vi "FL Generate 3D Graph.vi"(0 "Fuzzy Set In":T1 {"user MF interpolating polynomials"."coa_x(y) coeff" format="%.4g"; "user MF interpolating polynomials"."Area(y) coeff" format="%.4g"; "user MF interpolating polynomials"."X(y) coeff" format="%.4g"; "user MF interpolating polynomials"."Y(x) coeff" format="%.4g"; "user MF interpolating polynomials"."Y" format="%.4g"; "user MF interpolating polynomials"."X" format="%.4g"; "defuzzification method" items=["Center of Area", "Modified Center of Area", "Center of Sums", "Center of Maximum", "Mean of Maximum"]; "rules"."consequents"."Var Index" min=0; "rules"."consequents"."Cond" items=["=", "!="]; "rules"."consequents"."MF Index" min=0; "rules"."antecedents"."Var Index" min=0; "rules"."antecedents"."Cond" items=["=", "!="]; "rules"."antecedents"."MF Index" min=0; "rules"."consequent implication" items=["Minimum", "Product"]; "rules"."antecedent connective" items=["AND (Minimum)", "AND (Product)", "OR (Maximum)", "OR (Probabilistic)"]; "output variables"."MFs"."shape" items=["Triangle", "Trapezoid", "Singleton", "Sigmoid", "Gaussian", "User-Defined"]; "input variables"."MFs"."shape" items=["Triangle", "Trapezoid", "Singleton", "Sigmoid", "Gaussian", "User-Defined"]}, 1 "Input":dbl[](array[numeric]), 5 "Input Selection 1":i32, 7 "Input Selection 2":i32=1, 9 "Output":i32, 11 "error in (no error)":errorcluster, 12 "number of samples 1":i32=20, 13 "number of samples 2":i32=20) -> (4 "x":dbl[](array[numeric]), 6 "y":dbl[](array[numeric]), 10 "z":dbl[][](array[numeric]), 15 "error out":errorcluster)   [LabVIEW 2017, in "NI_Fuzzy_Logic_API.lvlib"]
uses:
  <vilib>/addons/Fuzzy Logic/NI_Fuzzy_Logic_API.lvlib
  <vilib>/addons/Fuzzy Logic/TypeDefs/FL System.ctl
  <vilib>/addons/Fuzzy Logic/TypeDefs/FL Variable.ctl
  <vilib>/addons/Fuzzy Logic/TypeDefs/FL Membership Function.ctl
  <vilib>/addons/Fuzzy Logic/TypeDefs/FL Membership Function Shape.ctl
  <vilib>/addons/Fuzzy Logic/TypeDefs/FL Rule.ctl
  <vilib>/addons/Fuzzy Logic/TypeDefs/FL Antecedent.ctl
  <vilib>/addons/Fuzzy Logic/TypeDefs/FL Modifier.ctl
  <vilib>/addons/Fuzzy Logic/TypeDefs/FL Antecedent Connective.ctl
  <vilib>/addons/Fuzzy Logic/TypeDefs/FL Consequent.ctl
  <vilib>/addons/Fuzzy Logic/TypeDefs/FL Consequent Implication.ctl
  <vilib>/addons/Fuzzy Logic/TypeDefs/FL Defuzzification.ctl
  <vilib>/addons/Fuzzy Logic/TypeDefs/FL Interpolating polynomials.ctl
  <vilib>/Analysis/1siggen.llb/Ramp Pattern by Samples.vi
  <vilib>/addons/Fuzzy Logic/FL Fuzzy Controller (MIMO).vi
  <vilib>/Analysis/NI_AALBase.lvlib
panel:
  # "IF"
  # "THEN"
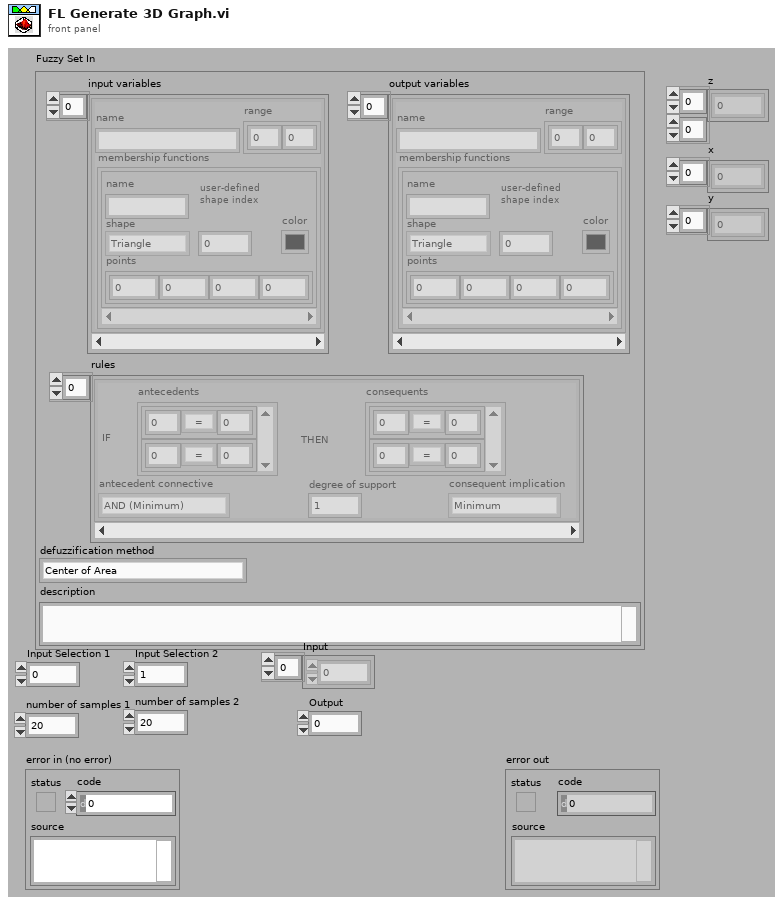
[diagram p1: front panel]
types:
  T1 = typedef "NI_Fuzzy_Logic_API.lvlib/FL System.ctl" = cluster{"input variables":T2[], "output variables":T2[], "rules":T5[], "defuzzification method":T11, "description":string, "user MF interpolating polynomials":T12[]}
  T2 = typedef "NI_Fuzzy_Logic_API.lvlib/FL Variable.ctl" = cluster{"name":string, "range":dbl[], "MFs":T3[]}
  T3 = typedef "NI_Fuzzy_Logic_API.lvlib/FL Membership Function.ctl" = cluster{"name":string, "shape":T4, "points":dbl[], "color":u32, "user-defined shape index":i32}
  T4 = typedef "NI_Fuzzy_Logic_API.lvlib/FL Membership Function Shape.ctl" = u16
  T5 = typedef "NI_Fuzzy_Logic_API.lvlib/FL Rule.ctl" = cluster{"antecedents":T6[], "antecedent connective":T8, "consequents":T9[], "consequent implication":T10, "degree of support":dbl}
  T6 = typedef "NI_Fuzzy_Logic_API.lvlib/FL Antecedent.ctl" = cluster{"Var Index":i32, "MF Index":i32, "Cond":T7}
  T7 = typedef "NI_Fuzzy_Logic_API.lvlib/FL Modifier.ctl" = u16
  T8 = typedef "NI_Fuzzy_Logic_API.lvlib/FL Antecedent Connective.ctl" = u16
  T9 = typedef "NI_Fuzzy_Logic_API.lvlib/FL Consequent.ctl" = cluster{"Var Index":i32, "MF Index":i32, "Cond":T7}
  T10 = typedef "NI_Fuzzy_Logic_API.lvlib/FL Consequent Implication.ctl" = u16
  T11 = typedef "NI_Fuzzy_Logic_API.lvlib/FL Defuzzification.ctl" = u16
  T12 = typedef "NI_Fuzzy_Logic_API.lvlib/FL Interpolating polynomials.ctl" = cluster{"X":dbl[], "Y":dbl[], "Y(x) coeff":dbl[][], "X(y) coeff":dbl[][], "Area(y) coeff":dbl[][], "coa_x(y) coeff":dbl[][]}
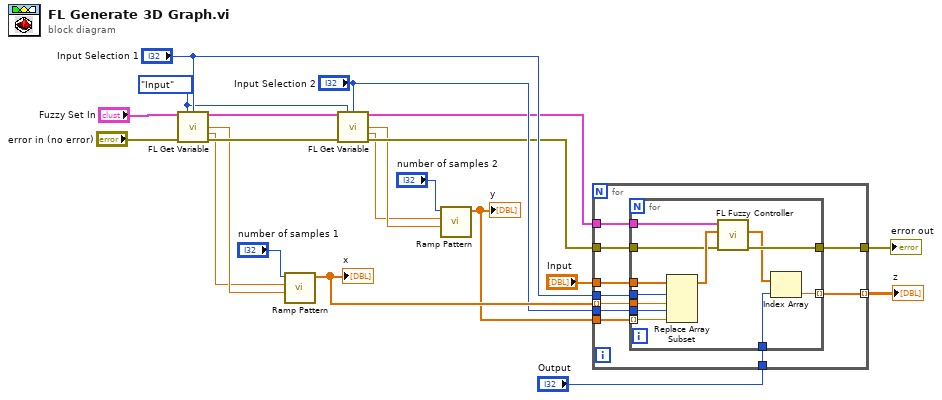
[diagram p0: block diagram]
diagram:
  w8 = enum16{"Input", "Output"}."Input" ("Input/Output")
  n1 = call <vilib>:"FL Get Variable.vi"("fuzzy system in"="Fuzzy Set In", "input/output"=w8, "variable index"="Input Selection 1", "error in (no error)"="error in (no error)") -> ("fuzzy system out"=w11:T1, "minimum"=w4:dbl, "maximum"=w3:dbl, "error out"=w9:errorcluster)  [unwired: 8 out]
  n2 = call-poly <vilib>:"Ramp Pattern.vi"("start"=w4, "end"=w3, "samples"="number of samples 1") -> ("Ramp Pattern"=w19:dbl[])  [unwired: 7 in, 1 out]
  "x" <- w19
  n3 = call <vilib>:"FL Get Variable.vi"("fuzzy system in"=w11, "input/output"=w8, "variable index"="Input Selection 2", "error in (no error)"=w9) -> ("fuzzy system out"=w10:T1, "minimum"=w2:dbl, "maximum"=w1:dbl, "error out"=w6:errorcluster)  [unwired: 8 out]
  n4 = call-poly <vilib>:"Ramp Pattern.vi"("start"=w2, "end"=w1, "samples"="number of samples 2") -> ("Ramp Pattern"=w16:dbl[])  [unwired: 7 in, 1 out]
  "y" <- w16
  n5 = for {
    tunnel: w19 -> [w31] mode=indexing
    tunnel: w16 -> [w30]
    tunnel: w10 -> [w29]
    tunnel: [w28] -> w17 mode=indexing
    tunnel: "Output" -> [w27]
    tunnel: "Input" -> [w26]
    tunnel: "Input Selection 2" -> [w25]
    tunnel: "Input Selection 1" -> [w24]
    tunnel: w6 -> [w23]
    tunnel: [w22] -> w5
    n6 = for {
      tunnel: w31 -> [w36]
      tunnel: w30 -> [w37] mode=indexing
      tunnel: w29 -> [w42]
      tunnel: [w41] -> w28 mode=indexing
      tunnel: w27 -> [w40]
      tunnel: w26 -> [w39]
      tunnel: w25 -> [w38]
      tunnel: w24 -> [w35]
      tunnel: w23 -> [w34]
      tunnel: [w33] -> w22
      n7 = Replace Array Subset(array=w39, new element #1=w36, index #1=w35, new element #2=w37, index #2=w38) -> (w43:dbl[])
      n8 = call-poly <vilib>:"FL Fuzzy Controller.vi"("error in (no error)"=w34, "input values"=w43, "fuzzy system in"=w42) -> ("error out"=w33:errorcluster, "output values"=w32:dbl[])  [unwired: 7 out]
      n9 = Index Array(array=w32, index=w40) -> (element=w41:dbl)
    }
  }
  "z" <- w17
  "error out" <- w5
